vi "PRIME Detector Read All Responses.vi"(7 "Log":bool, 8 "error in":errorcluster, 10 "Str Ref":refnum<vi>, 11 "connection ID":refnum<k5>) -> (0 "error out":errorcluster, 1 "Responses":string[](array[string]), 2 "Status Response":string, 3 "connection ID out":refnum<k5>)   [LabVIEW 2024, in "PRIME Detector.lvclass"]
uses:
  PRIME Detector.lvclass
  <vilib>/Utility/error.llb/Trim Whitespace One-Sided.vi
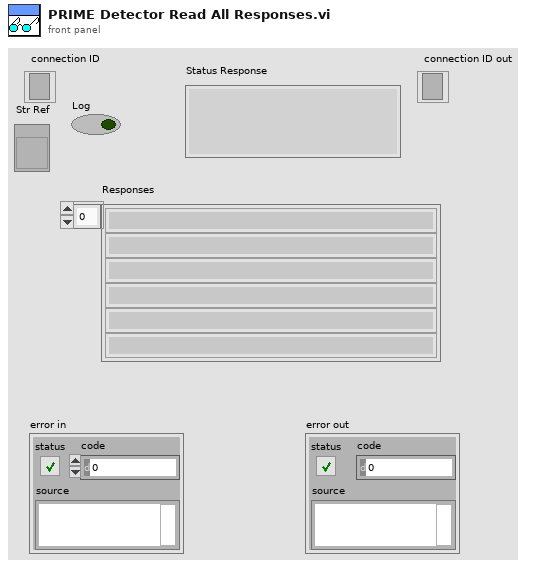
[diagram p1: front panel]
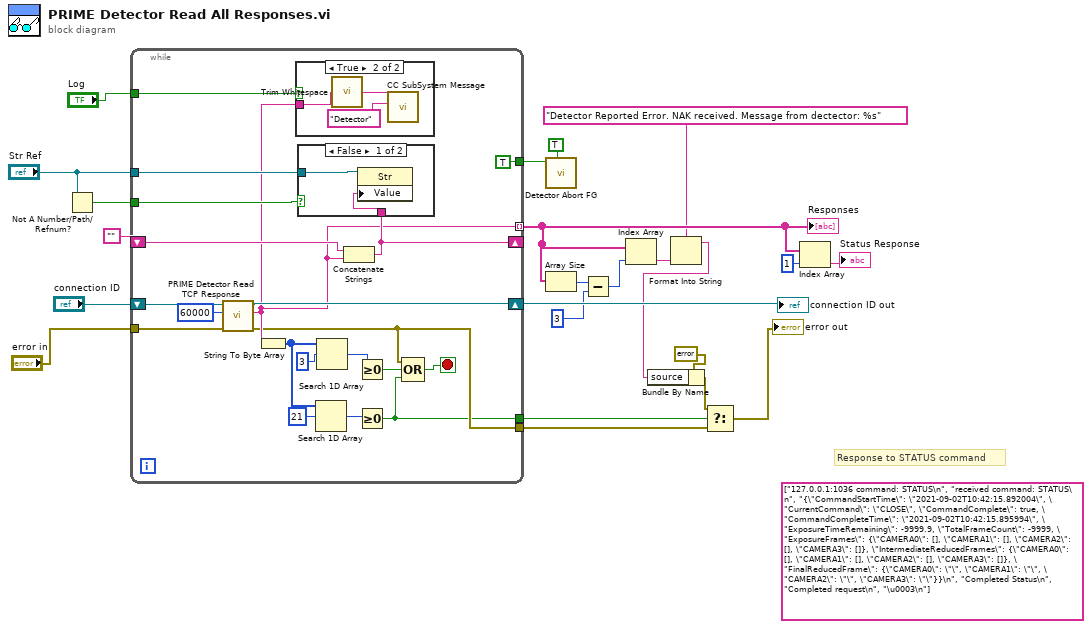
[diagram p0: block diagram]
diagram:
  (unwired) string[] ["127.0.0.1:1036 command: STATUS\n", "received command: STATUS\n", "{\"CommandStartTime\": \"2021-09-02T10:42:15.892004\", \"CurrentCommand\": \"CLOSE\", \"CommandComplete\": true, \"CommandCompleteTime\": \"2021-09-02T10:42:15.895994\", \"ExposureTimeRemaining\": -9999.9, \"TotalFrameCount\": -9999, \"ExposureFrames\": {\"CAMERA0\": [], \"CAMERA1\": [], \"CAMERA2\": [], \"CAMERA3\": []}, \"IntermediateReducedFrames\": {\"CAMERA0\": [], \"CAMERA1\": [], \"CAMERA2\": [], \"CAMERA3\": []}, \"FinalReducedFrame\": {\"CAMERA0\": \"\", \"CAMERA1\": \"\", \"CAMERA2\": \"\", \"CAMERA3\": \"\"}}\n", "Completed Status\n", "Completed request\n", "\u0003\n"] ("Responses")
  # "Response to STATUS command"
  n1 = Not A Number/Path/Refnum?(number/path/refnum="Str Ref") -> (NaN/Path/Refnum?=w18:bool)
  n2 = while {
    tunnel: "error in" -> [w42]
    tunnel: [w30] -> w9 mode=indexing
    shift-right: [w41] -> w19
    shift-left: "connection ID" -> [w43]
    tunnel: w18 -> [w35]
    tunnel: "Str Ref" -> [w34]
    shift-right: [w32] -> _
    shift-left: "" -> [w33]
    tunnel: "Log" -> [w31]
    tunnel: [w26] -> w14
    tunnel: [w25] -> w13
    tunnel: [TRUE] -> w2
    stop <- w38 stop-if-true
    n3 = call "PRIME Detector Read TCP Response.vi"("error in (no error)"=w42, "timeout ms (6000)"=60000, "connection ID"=w43) -> ("error out"=w26:errorcluster, "response message"=w30:string, "connection ID out"=w41:refnum<k5>)  [unwired: 5 in, 1 out]
    n4 = String To Byte Array(string=w30) -> (unsigned byte array=w29:u8[])
    n5 = case shown="True" w31 {
      tunnel: w30 -> [_ w46]
      frame False {
      }
      frame True {
        n6 = call <vilib>:"Trim Whitespace.vi"("string"=w46) -> ("trimmed string"=w45:string)  [unwired: 1 in]
        n7 = call "CC SubSystem Message.vi"("Subsystem"="Detector", "Message"=w45) -> ()  [unwired: 9 in, 1 out]
      }
    }
    n8 = Search 1D Array(1D array=w29, element=u8 21) -> (index of element=w27:i32)  [unwired: 1 in]
    n9 = Search 1D Array(1D array=w29, element=u8 3 ("y")) -> (index of element=w40:i32)  [unwired: 1 in]
    n10 = Concatenate Strings(w33, w30) -> (w32:string)
    n11 = case shown="False" w35 {
      tunnel: w34 -> [w48 _]
      tunnel: w32 -> [w47 _]
      frame False {
        n12 = property class="Str"(reference=w48, "Value"=w47) -> ()  [unwired: 1 in, 2 out]
      }
      frame True {
      }
    }
    n13 = Greater Or Equal To 0?(x=w40) -> (x >= 0?=w39:bool)
    n14 = Greater Or Equal To 0?(x=w27) -> (x >= 0?=w25:bool)
    n15 = Compound Arithmetic op=OR(w26, w39, w25) -> (w38:bool)
  }
  "Responses" <- w9
  "connection ID out" <- w19
  n16 = call "Detector Abort FG.vi"("init"=TRUE, "state"=w2) -> ()  [unwired: 8 in, 2 out]
  n17 = Array Size(array=w9) -> (size(s)=w8:i32)
  n18 = Subtract(x=w8, y=3) -> (x-y=w3:i32)
  n19 = Index Array(array=w9, index=w3) -> (element=w5:string)
  n20 = Format Into String(format string="Detector Reported Error. NAK received. Message from dectector: %s" ("source"), w5) -> (resulting string=w4:string)  [unwired: 2 in, 1 out]
  n21 = Bundle By Name(cluster=errorcluster {"status"=TRUE, "code"=5000, "source"=""} ("t"), "source"=w4) -> (w10:errorcluster)
  n22 = Select(t=w10, s=w13, f=w14) -> (s? t:f=→"error out":errorcluster)
  n23 = Index Array(array=w9, index=1) -> (element=→"Status Response":string)
